vi "Write Go-NoGo GUID.vi"(8 "error in (no error)":errorcluster, 10 "Go-NoGo GUID":string, 11 "Ancestor in":refnum<class "Ancestor.lvclass">) -> (0 "error out":errorcluster, 3 "Ancestor out":refnum<class "Ancestor.lvclass">)   [LabVIEW 2026, in "TALOS.lvlib" / "Ancestor.lvlib" / "Ancestor.lvclass"]
uses:
  Ancestor.lvclass
  Ancestor.lvclass/Ancestor.ctl
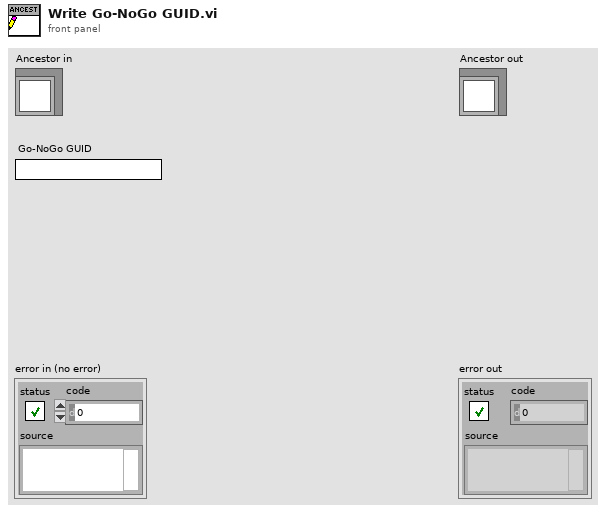
[diagram p1: front panel]
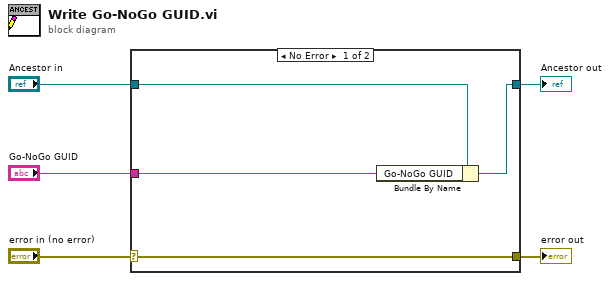
[diagram p0: block diagram]
diagram:
  n1 = case shown="No Error" "error in (no error)" {
    selector: "error in (no error)" -> [w9 w10]
    tunnel: [w9 w10] -> w4
    tunnel: [w7 w11] -> w2
    tunnel: "Ancestor in" -> [w8 w11]
    tunnel: "Go-NoGo GUID" -> [w6 _]
    frame No Error {
      n2 = Bundle By Name(cluster=w8, "Go-NoGo GUID"=w6) -> (w7:refnum<class "Ancestor.lvclass">)
    }
    frame Error {
    }
  }
  "error out" <- w4
  "Ancestor out" <- w2
